vi "Program_Load_v02.vi"(8 "error in (no error)":errorcluster, 9 "Time Start":dbl[unit], 10 "Program Spin Coater":T1(array[cluster]), 11 "SpinCoater in":refnum<class "SpinCoater.lvclass">) -> (0 "error out":errorcluster, 3 "SpinCoater out":refnum<class "SpinCoater.lvclass">)   [LabVIEW 2020, in "SpinCoater.lvclass"]
uses:
  <instrlib>/Classes/SpinCoater/SpinCoater.lvclass
panel:
  out "read buffer":string
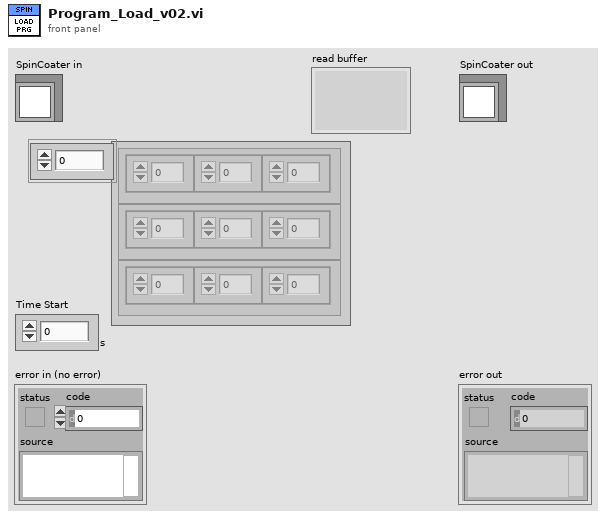
[diagram p1: front panel]
types:
  T1 = cluster{"Speed (rpm)":dbl, "Time (s)":dbl, "Acc (rpm/s)":dbl}[]
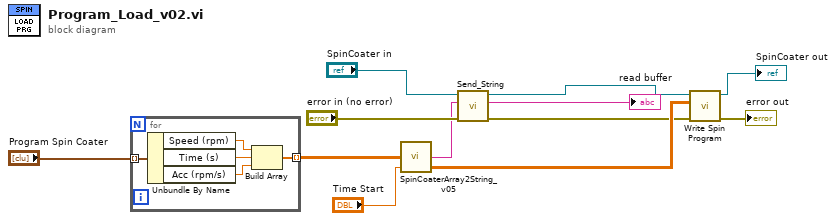
[diagram p0: block diagram]
diagram:
  n1 = for {
    tunnel: "Program Spin Coater" -> [w17] mode=indexing
    tunnel: [w13] -> w4 mode=indexing
    n2 = Unbundle By Name(w17) -> ("Speed (rpm)"=w16:dbl, "Time (s)"=w15:dbl, "Acc (rpm/s)"=w14:dbl)
    n3 = Build Array(w16, w15, w14) -> (w13:dbl[])
  }
  n4 = call <instrlib>:"SpinCoaterArray2String_v05.vi"("Time Start"="Time Start", "Program Spin Coater\nSpeed (rpm)          Time (s)"=w4) -> ("Prg Spin Coater small"=w8:dbl[][], "remote control String"=w9:string)  [unwired: 2 in]
  n5 = call-dynamic "Send_String.vi"("error in (no error)"="error in (no error)", "String"=w9, "SpinCoater in"="SpinCoater in") -> ("error out"=w3:errorcluster, "read buffer"=→"read buffer":string, "SpinCoater out"=w1:refnum<class "SpinCoater.lvclass">)  [unwired: 6 in]
  n6 = call-dynamic "Write Spin Program.vi"("error in (no error)"=w3, "Spin Program"=w8, "SpinCoater in"=w1) -> ("error out"=→"error out":errorcluster, "SpinCoater out"=→"SpinCoater out":refnum<class "SpinCoater.lvclass">)  [unwired: 7 in]
